vi "JSON Tree to Name.vi"(8 "error in (no error)":errorcluster, 11 "JSON Array":variant) -> (0 "error out":errorcluster, 2 "Name":string, 3 "JSON Tree Out Passthrough":variant)   [LabVIEW 2015, in "SLSC Switch.lvlib" / "SLSC Switch.lvclass"]
uses:
  SLSC Switch.lvclass
  <vilib>/LVH/i3 JSON/JSON Parsing/Get Object Parameter Files/Get Object Parameter - String.vi
  <vilib>/LVH/i3 JSON/i3-json.lvlib
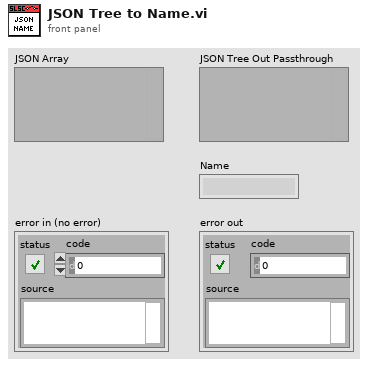
[diagram p1: front panel]
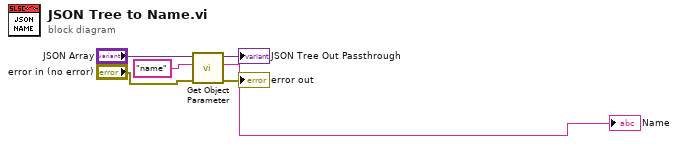
[diagram p0: block diagram]
diagram:
  n1 = call-poly <vilib>:"Get Object Parameter.vi"("error in (no error)"="error in (no error)", "Parameter Name"="name", "JSON Tree In (JSON Object)"="JSON Array") -> ("error out"=→"error out":errorcluster, "String Value"=→"Name":string, "JSON Tree Out Passthrough"=→"JSON Tree Out Passthrough":variant)  [unwired: 5 in, 1 out]
